vi "cRIO_FPGA_COMMUNICATION Behandle FPGA Schreibe Daten.vi"(8 "Station":bool[](array[boolean])=[FALSE, FALSE, FALSE, FALSE, FALSE, FALSE, FALSE, FALSE], 9 "Band":bool[](array[boolean])=[FALSE, FALSE, FALSE, FALSE, FALSE, FALSE, FALSE, FALSE], 10 "Station Index":T2, 11 "FGV Band/Station Commands":T1=enum."Schreibe") -> (2 "Stationen":bool[][](array[boolean]), 3 "Bänder":bool[][](array[boolean]))   [LabVIEW 2013, in "cRIO_FPGA_COMMUNICATION.lvlib"]
uses:
  cRIO_FPGA_COMMUNICATION.lvlib
  TYPES/TYPE Station Index.ctl
  TYPES/TYPE Band und Stations Kommandos.ctl
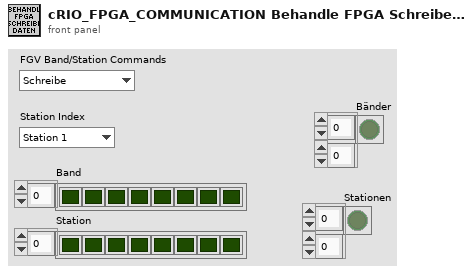
[diagram p1: front panel]
types:
  T1 = typedef "cRIO_FPGA_COMMUNICATION.lvlib/TYPE Band und Stations Kommandos.ctl" = enum16{"Init", "Lese", "Schreibe"}
  T2 = typedef "cRIO_FPGA_COMMUNICATION.lvlib/TYPE Station Index.ctl" = enum16{"Station 1", "Station 2", "Station 3", "Station 4", "Station 5", "Station 6", "Station 7", "Station 8", "Station 9", "Station 10", "Station 11", "Station 12", "Station 13", "Station 14", "Station 15", "Station 16", "Station 17", "Station 18", "Station 19", "Station 20"}
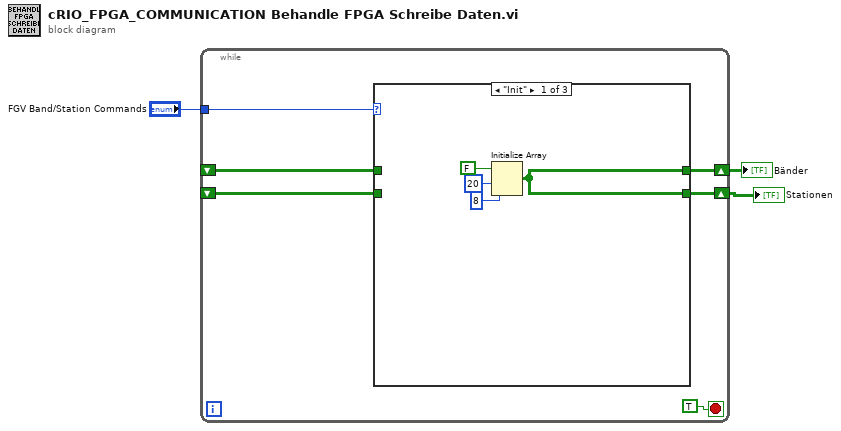
[diagram p0: block diagram]
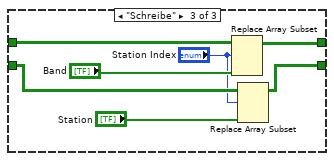
[diagram p3: hidden frame]
diagram:
  n1 = while {
    tunnel: "FGV Band/Station Commands" -> [w8]
    shift-right: [w7] -> w2
    shift-left: _ -> [w6]
    shift-right: [w5] -> w1
    shift-left: _ -> [w4]
    stop <- TRUE stop-if-true
    n2 = case shown="\"Init\"" w8 {
      tunnel: [w10 w15 w21] -> w7
      tunnel: w6 -> [_ w15 w22]
      tunnel: [w10 w14 w19] -> w5
      tunnel: w4 -> [_ w14 w20]
      frame "Init" {
        n3 = Initialize Array(FALSE, 20 ("Dimension"), 8 ("Dimension")) -> (w10:bool[][])
      }
      frame "Lese" {
      }
      frame "Schreibe" {
        n4 = Replace Array Subset(array=w22, new element="Band", index (row)="Station Index") -> (w21:bool[][])  [unwired: 1 in]
        n5 = Replace Array Subset(array=w20, new element="Station", index (row)="Station Index") -> (w19:bool[][])  [unwired: 1 in]
      }
    }
  }
  "Bänder" <- w2
  "Stationen" <- w1
